vi "Fetch Waveform.vi"(8 "error in":errorcluster, 10 "Channel":i32, 11 "OWON SDS1022 in":refnum<class "OWON SDS1022.lvclass">) -> (0 "error out":errorcluster, 3 "OWON SDS1022 out":refnum<class "OWON SDS1022.lvclass">)   [LabVIEW 2023, in "OWON SDS1022.lvclass"]
doc: "Since more than one Channel could be configured for Acquisition one has to specify\nwhich specific channel data to fetch"
uses:
  OWON SDS1022.lvclass
  OWON SDS1022.lvclass/OWON SDS1022.ctl
  HAL/Scope Base/Scope Base.lvclass/Scope Base.ctl
  <vilib>/JDP Science/JSONtext/Find Item.vi
  <vilib>/JDP Science/JSONtext/Next JSON Value.vi
  <vilib>/JDP Science/JSONtext/String Subset.vi
  <vilib>/JDP Science/JSONtext/Parsing/Advance past next JSON Value (inlined COPY).vi
  <vilib>/JDP Science/JSONtext/Parsing/Advance past whitespace.vi
  <vilib>/JDP Science/JSONtext/Parsing/Advance past String.vi
  <vilib>/JDP Science/JSONtext/Parsing/Advance past Number.vi
  <vilib>/JDP Science/JSONtext/Parsing/Advance past Line Ending.vi
  <vilib>/JDP Science/JSONtext/Parsing/Parse Full Path or Item Name.vi
  <vilib>/JDP Science/JSONtext/Parsing/Advance past Array.vi
  <vilib>/JDP Science/JSONtext/Parsing/Advance past Object.vi
  <vilib>/JDP Science/JSONtext/support/Error Cluster From Code.vi
  <vilib>/JDP Science/JSONtext/Offset/Find Item Locations by Path.vi
  <vilib>/JDP Science/JSONtext/JSON text to Variant.vi
  <vilib>/Utility/error.llb/Error Cluster From Error Code.vi
  <vilib>/JDP Science/JSONtext/LVClass Serializer/JSONtext LVClass Serializer.lvclass
  <vilib>/ErrorRing/Error Ring.xnode
panel:
  out "Fetched Points":i16[](graph)
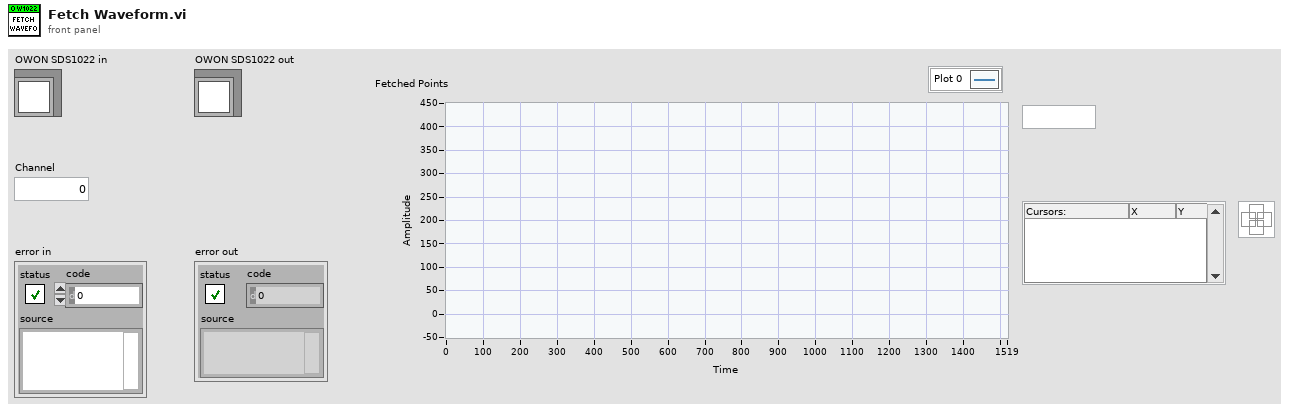
[diagram p1: front panel]
types:
  T1 = enum16{"big-endian, network order", "native, host order", "little-endian"}
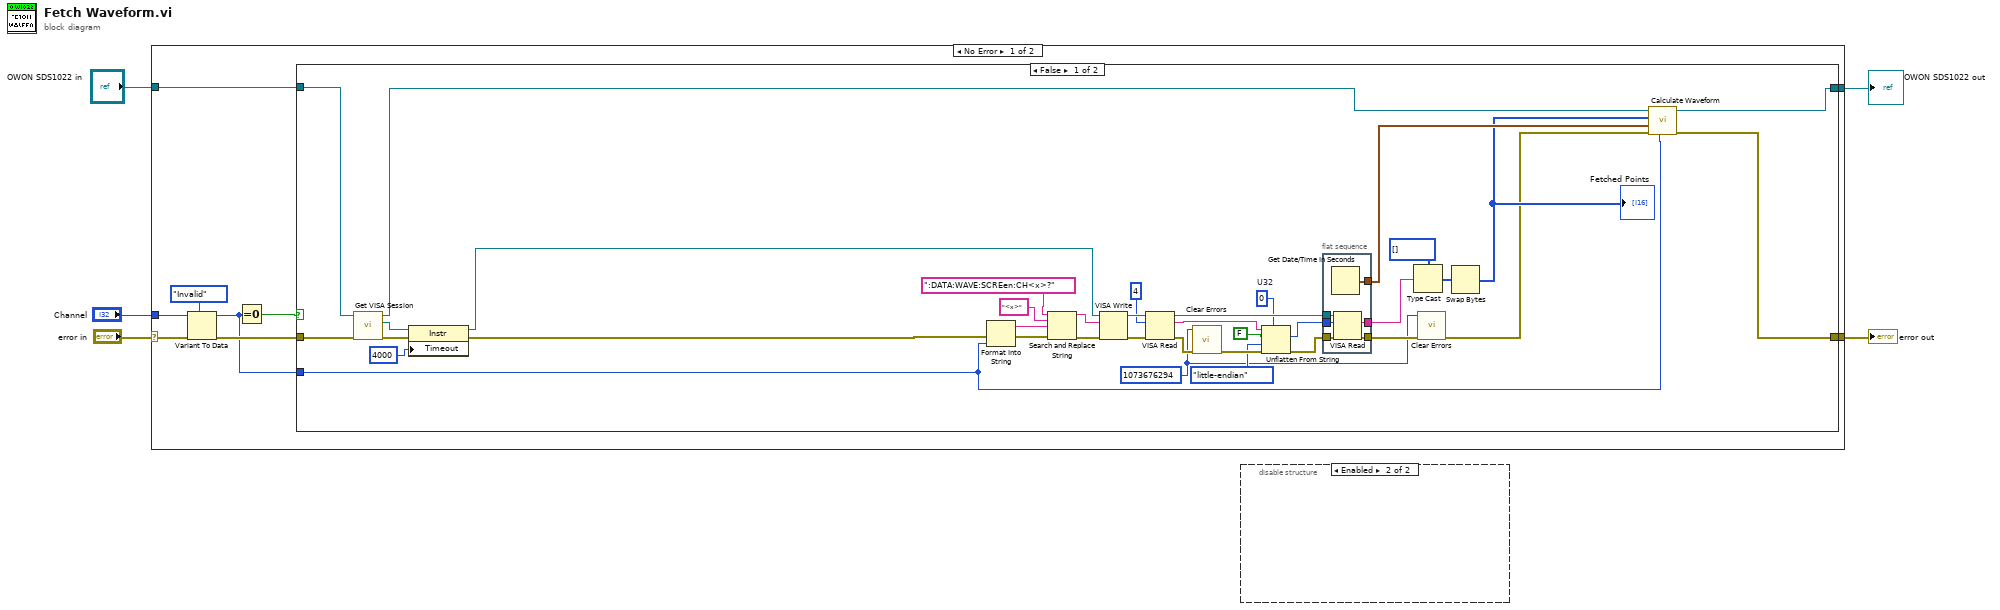
[diagram p0: block diagram]
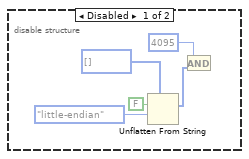
[diagram p2: hidden frame]
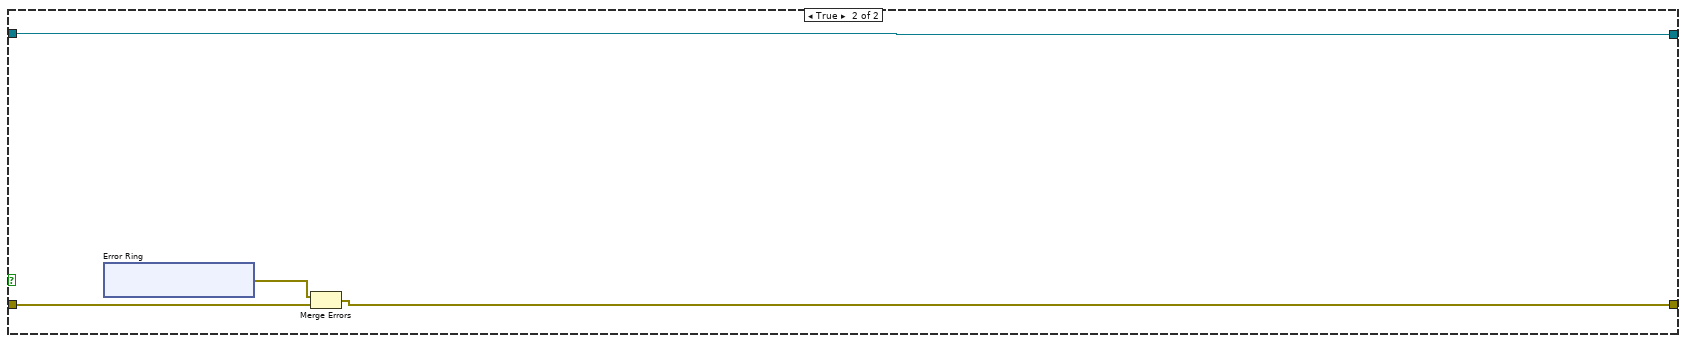
[diagram p3: hidden frame]
diagram:
  n1 = case shown="No Error" "error in" {
    selector: "error in" -> [w8 w68]
    tunnel: "OWON SDS1022 in" -> [w14 w67]
    tunnel: [w13 w67] -> w4
    tunnel: [w12 w68] -> w3
    tunnel: "Channel" -> [w10 _]
    frame No Error {
      n2 = Variant To Data(error in=w8, type=enum16{"Invalid", "Channel 1", "Channel 2"}."Invalid" ("Channel"), Variant=w10) -> (data=w6:enum16{"Invalid", "Channel 1", "Channel 2"}, error out=w7:errorcluster)
      n3 = Equal To 0?(x=w6) -> (x = 0?=w9:bool)
      n4 = case shown="False" w9 {
        tunnel: w14 -> [w32 w58]
        tunnel: [w20 w58] -> w13
        tunnel: [w16 w59] -> w12
        tunnel: w7 -> [w31 w60]
        tunnel: w6 -> [w15 _]
        frame False {
          w29 = 1073676294 ("specific error code to clear (0: all)")
          w34 = u32 0  # U32
          n5 = call-dynamic "Get VISA Session.vi"("error in"=w31, "Scope VISA in"=w32) -> ("error out"=w30:errorcluster, "VISA session"=w28:refnum<visa-resource-name>, "Scope VISA out"=w21:refnum<class "OWON SDS1022.lvclass">)  [unwired: 7 in]
          n6 = property class="Instr"(reference=w28, error in=w30, "Timeout"=u32 4000 ("General Settings:Timeout Value")) -> (reference out=w22:refnum<visa-resource-name>, error out=w23:errorcluster)
          n7 = Format Into String(error in=w23, w15) -> (resulting string=w47:string, error out=w48:errorcluster)  [unwired: 2 in]
          n8 = Search and Replace String(input string=":DATA:WAVE:SCREen:CH<x>?" ("write buffer"), search string="<x>", replace string=w47, error in=w48) -> (result string=w46:string, error out=w45:errorcluster)  [unwired: 4 in, 2 out]
          n9 = VISA Write(VISA resource name=w22, write buffer=w46, error in (no error)=w45) -> (VISA resource name out=w43:refnum<visa-resource-name>, error out=w51:errorcluster)  [unwired: 1 out]
          n10 = VISA Read(VISA resource name=w43, byte count=u32 4, error in (no error)=w51) -> (VISA resource name out=w42:refnum<visa-resource-name>, read buffer=w35:string, error out=w44:errorcluster)  [unwired: 1 out]
          n11 = call <vilib>:"Clear Errors.vi"("error in (no error)"=w44, "specific error code to clear (0: all)"=w29) -> ("error out"=w39:errorcluster)  [unwired: 4 in, 1 out]
          n12 = Unflatten From String(type=w34, binary string=w35, data includes array or string size? (T)=FALSE, byte order (0:big-endian, network order)=T1."little-endian", error in (no error)=w39) -> (value=w33:u32, error out=w38:errorcluster)  [unwired: 1 out]
          n13 = flat-sequence {
            tunnel: w42 -> [w57]
            tunnel: [w56] -> w40
            tunnel: w38 -> [w55]
            tunnel: w33 -> [w54]
            tunnel: [w53] -> w26
            tunnel: [w52] -> w19
            frame #0 {
              n14 = Get Date/Time In Seconds() -> (seconds since 1Jan1904=w52:timestamp)
              n15 = VISA Read(VISA resource name=w57, byte count=w54, error in (no error)=w55) -> (read buffer=w53:string, error out=w56:errorcluster)  [unwired: 2 out]
            }
          }
          n16 = Type Cast(type=i16[] [], x=w26) -> (*(type *) &x=w24:i16[])
          n17 = call <vilib>:"Clear Errors.vi"("error in (no error)"=w40, "specific error code to clear (0: all)"=w29) -> ("error out"=w17:errorcluster)  [unwired: 4 in, 1 out]
          n18 = Swap Bytes(anything=w24) -> (byte swapped=w18:i16[])
          "Fetched Points" <- w18
          n19 = call "Calculate Waveform.vi"("Channel"=w15, "error in (no error)"=w17, "Acquisition Time"=w19, "Points"=w18, "OWON SDS1022 in"=w21) -> ("error out"=w16:errorcluster, "OWON SDS1022 out"=w20:refnum<class "OWON SDS1022.lvclass">)  [unwired: 5 in]
        }
        frame True {
          n20 = xnode "Error Ring"() -> ("error out"=w61:errorcluster)
          n21 = Merge Errors(w61, w60) -> (w59:errorcluster)
        }
      }
    }
    frame Error {
    }
  }
  "error out" <- w3
  "OWON SDS1022 out" <- w4
  n22 = disable-structure shown="Enabled" {
    frame Disabled {
      n23 = Unflatten From String(type=i16[] [], data includes array or string size? (T)=FALSE, byte order (0:big-endian, network order)=T1."little-endian") -> (value=w73:i16[])  [unwired: 2 in, 2 out]
      n24 = And(x=4095, y=w73) -> ()  [unwired: 1 out]
    }
    frame Enabled {
    }
  }
